vi "Set Time Stamp.vi"(8 "error in (no error)":errorcluster, 10 "Time Stamp":timestamp format="%<%x %.3X>T", 11 "CAN Message in":refnum<class "CAN Message.lvclass">) -> (0 "error out":errorcluster, 3 "CAN Message out":refnum<class "CAN Message.lvclass">)   [LabVIEW 2024, in "PCAN.lvlib" / "CAN Message.lvclass"]
uses:
  CAN Message.lvclass
  CAN Message.lvclass/CAN Message.ctl
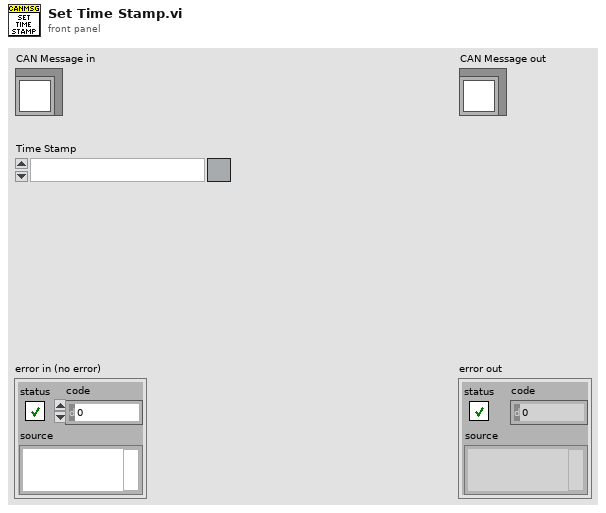
[diagram p1: front panel]
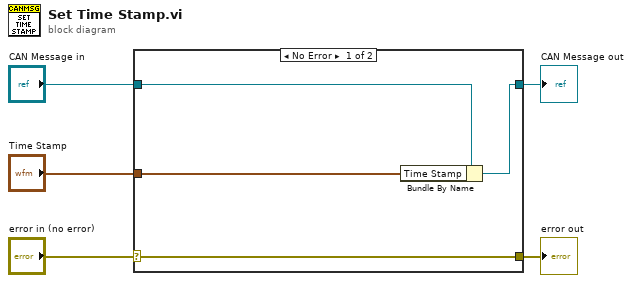
[diagram p0: block diagram]
diagram:
  n1 = case shown="No Error" "error in (no error)" {
    selector: "error in (no error)" -> [w9 w10]
    tunnel: [w9 w10] -> w4
    tunnel: [w7 w11] -> w2
    tunnel: "CAN Message in" -> [w8 w11]
    tunnel: "Time Stamp" -> [w6 _]
    frame No Error {
      n2 = Bundle By Name(cluster=w8, "Time Stamp"=w6) -> (w7:refnum<class "CAN Message.lvclass">)
    }
    frame Error {
    }
  }
  "error out" <- w4
  "CAN Message out" <- w2
